vi "Step3-1.vi"(1 "cluster":i32, 2 "n":i32=2, 3 "v":dbl[](array[numeric]), 4 "X":dbl[][](array[numeric])) -> (0 "Array":dbl[][](array[numeric]))   [LabVIEW 2011]
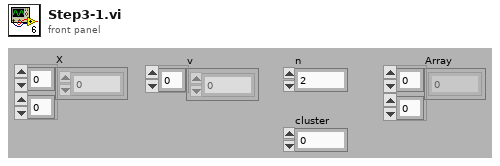
[diagram p1: front panel]
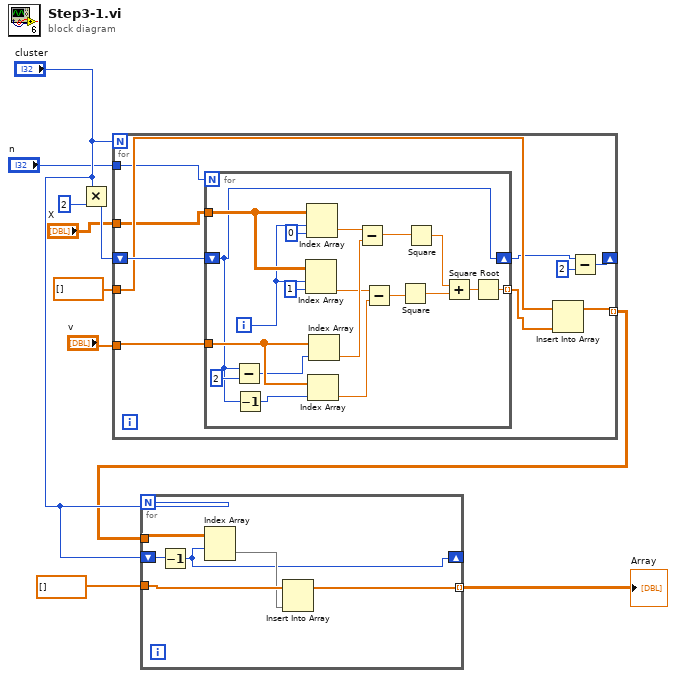
[diagram p0: block diagram]
diagram:
  n1 = Multiply(x="cluster", y=2) -> (x*y=w5:i32)
  n2 = for {
    N: "cluster" -> [_]
    shift-right: [w14] -> _
    shift-left: w5 -> [w20]
    tunnel: [w17] -> w7 mode=indexing
    tunnel: dbl[] [] -> [w18]
    tunnel: "v" -> [w13]
    tunnel: "X" -> [w12]
    tunnel: "n" -> [w11]
    n3 = for {
      N: w11 -> [_]
      tunnel: w12 -> [w39]
      tunnel: w13 -> [w35]
      tunnel: [w25] -> w19 mode=indexing
      shift-right: [w21] -> w16
      shift-left: w20 -> [w21]
      i -> [w38]
      n4 = Subtract(x=w21, y=2) -> (x-y=w22:i32)
      n5 = Decrement(x=w21) -> (x-1=w23:i32)
      n6 = Index Array(array=w39, index (row)=w38, index (col)=1 ("disabled index (col)")) -> (element=w31:dbl)
      n7 = Index Array(array=w39, index (row)=w38, index (col)=0 ("disabled index (col)")) -> (element=w34:dbl)
      n8 = Index Array(array=w35, index=w23) -> (element=w30:dbl)
      n9 = Index Array(array=w35, index=w22) -> (element=w33:dbl)
      n10 = Subtract(x=w34, y=w33) -> (x-y=w32:dbl)
      n11 = Subtract(x=w31, y=w30) -> (x-y=w29:dbl)
      n12 = Square(x=w29) -> (x^2=w28:dbl)
      n13 = Square(x=w32) -> (x^2=w27:dbl)
      n14 = Add(x=w27, y=w28) -> (x+y=w26:dbl)
      n15 = Square Root(x=w26) -> (sqrt(x)=w25:dbl)
    }
    n16 = Insert Into Array(array=w18, new element=w19) -> (w17:dbl[])  [unwired: 1 in]
    n17 = Subtract(x=w16, y=2) -> (x-y=w14:i32)
  }
  n18 = for {
    N: "cluster" -> [_]
    tunnel: dbl[] [] -> [w45]
    tunnel: w7 -> [w44]
    shift-right: [w40] -> _
    shift-left: "cluster" -> [w43]
    tunnel: [w41] -> w10 mode=indexing
    n19 = Decrement(x=w43) -> (x-1=w40:i32)
    n20 = Index Array(array=w44, index (row)=w40) -> (element=w42:dbl[])  [unwired: 1 in]
    n21 = Insert Into Array(array=w45, new element=w42) -> (w41:dbl[])  [unwired: 1 in]
  }
  "Array" <- w10
